vi "SetScale.vi"(0 "max":dbl format="%.2f", 1 "min":dbl format="%.2f", 2 "Active Y Scale":i32, 3 "reference":refnum<vi>) -> ()   [LabVIEW 2009]
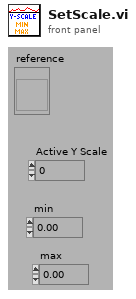
[diagram p1: front panel]
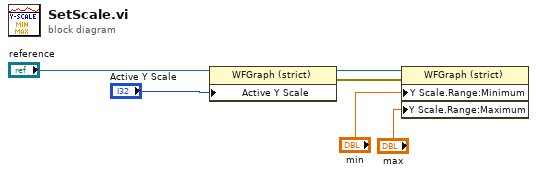
[diagram p0: block diagram]
diagram:
  n1 = property on="Property Node" class="WFGraph (strict)"(reference="reference", "Active Y Scale"="Active Y Scale") -> (error out=w3:errorcluster)  [unwired: 1 in, 1 out]
  n2 = property on="Property Node" class="WFGraph (strict)"(reference="reference", error in=w3, "Y Scale.Range:Minimum"="min", "Y Scale.Range:Maximum"="max") -> ()  [unwired: 2 out]
